vi "Post-Process.vi"(11 "Main Controller Actor in":refnum<class "Main Controller Actor.lvclass">) -> (3 "Main Controller Actor out":refnum<class "Main Controller Actor.lvclass">)   [LabVIEW 2021, in "Main Controller Actor.lvclass"]
uses:
  Main Controller Actor.lvclass
  Main Controller Actor.lvclass/Main Controller Actor.ctl
  Element/Element.lvclass
  Globals.vi
  5200b562-32ad-491b-9c97-f0d2b317c967.vi
  fb94a685-9cbf-46d1-b0f8-8938b087fb03.vi
panel:
  out "size(s)":i32
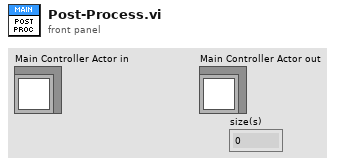
[diagram p1: front panel]
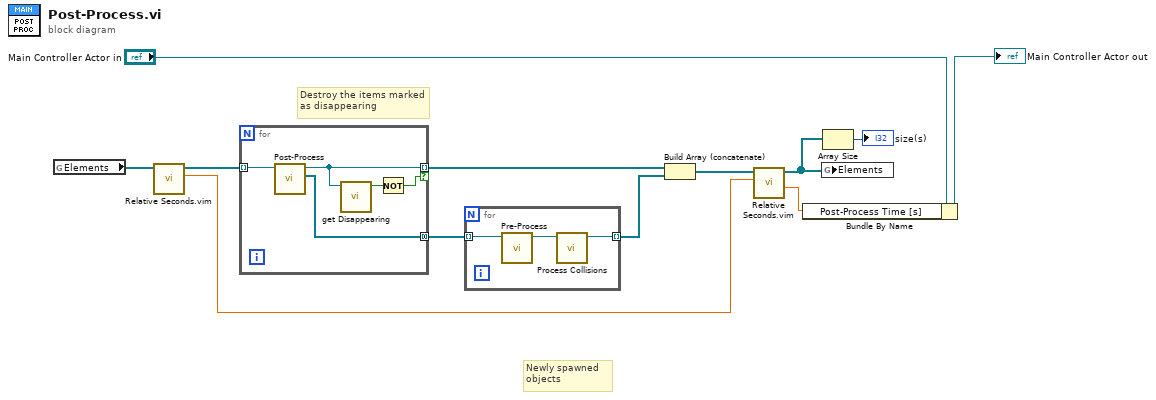
[diagram p0: block diagram]
diagram:
  # "Newly spawned objects"
  # "Destroy the items marked as disappearing"
  n1 = global read "Globals.vi" "Elements"() -> (w10:refnum<class "Element.lvclass">[])
  n2 = call "Relative Seconds.vim"("Anything in"=w10) -> ("Relative Seconds out"=w5:dbl, "Anything out"=w9:refnum<class "Element.lvclass">[])  [unwired: 8 in, 1 out]
  n3 = for {
    tunnel: [w15] -> w8 mode=indexing if=w14
    tunnel: w9 -> [w17] mode=indexing
    tunnel: [w16] -> w3 mode=concatenating
    n4 = call-dynamic "Post-Process.vi"("Element in"=w17) -> ("New Elements"=w16:refnum<class "Element.lvclass">[], "Element out"=w15:refnum<class "Element.lvclass">)  [unwired: 9 in]
    n5 = call "get Disappearing.vi"("Element in"=w15) -> ("Disappearing"=w13:bool)  [unwired: 10 in]
    n6 = Not(x=w13) -> (.not. x?=w14:bool)
  }
  n7 = for {
    tunnel: [w18] -> w2 mode=indexing
    tunnel: w3 -> [w20] mode=indexing
    n8 = call-dynamic "Pre-Process.vi"("Element in"=w20) -> ("Element out"=w19:refnum<class "Element.lvclass">)  [unwired: 10 in]
    n9 = call-dynamic "Process Collisions.vi"("Element in"=w19) -> ("Element out"=w18:refnum<class "Element.lvclass">)  [unwired: 10 in]
  }
  n10 = Build Array (concatenate)(w8, w2) -> (w7:refnum<class "Element.lvclass">[])
  n11 = call "Relative Seconds.vim"("Relative Seconds in"=w5, "Anything in"=w7) -> ("Relative Seconds delta"=w4:dbl, "Anything out"=w6:refnum<class "Element.lvclass">[])  [unwired: 7 in, 1 out]
  n12 = Bundle By Name(cluster="Main Controller Actor in", "Post-Process Time [s]"=w4) -> (→"Main Controller Actor out":refnum<class "Main Controller Actor.lvclass">)
  n13 = global write "Globals.vi" "Elements"(w6) -> ()
  n14 = Array Size(array=w6) -> (size(s)=→"size(s)":i32)
